vi "Step Association Retrieve Record.vi"(8 "error in (no error)":errorcluster, 11 "Statement Refnum":T1) -> (0 "error out":errorcluster, 2 "Association":T2, 3 "Statement Refnum":T1)   [LabVIEW 2011]
uses:
  Step Association Record.ctl
  SI.LIB/ODBC/SQL Controls/Statement Refnum.ctl
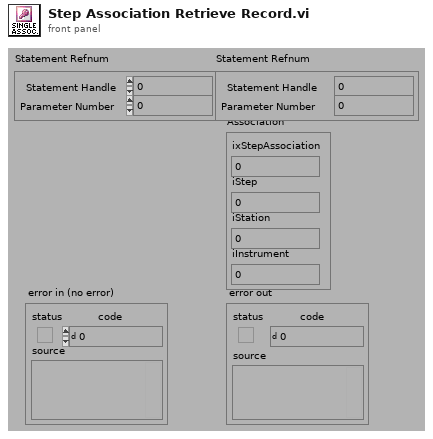
[diagram p1: front panel]
types:
  T1 = typedef "Statement Refnum.ctl" = cluster{"Statement Handle":i32, "Parameter Number":u16}
  T2 = typedef "Step Association Record.ctl" = cluster{"ixStepAssociation":i32, "iStep":i32, "iStation":i32, "iInstrument":i32}
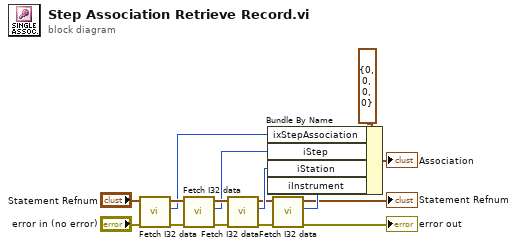
[diagram p0: block diagram]
diagram:
  n1 = call "Fetch I32 data.vi"("error in (no error)"="error in (no error)", "Statement Refnum"="Statement Refnum") -> ("error out"=w14:errorcluster, "Data"=w10:i32, "Statement Refnum"=w13:T1)  [unwired: 3 out]
  n2 = call "Fetch I32 data.vi"("error in (no error)"=w14, "Statement Refnum"=w13) -> ("error out"=w11:errorcluster, "Data"=w9:i32, "Statement Refnum"=w12:T1)  [unwired: 3 out]
  n3 = call "Fetch I32 data.vi"("error in (no error)"=w11, "Statement Refnum"=w12) -> ("error out"=w1:errorcluster, "Data"=w8:i32, "Statement Refnum"=w2:T1)  [unwired: 3 out]
  n4 = call "Fetch I32 data.vi"("error in (no error)"=w1, "Statement Refnum"=w2) -> ("error out"=→"error out":errorcluster, "Data"=w5:i32, "Statement Refnum"=→"Statement Refnum":T1)  [unwired: 3 out]
  n5 = Bundle By Name(cluster=T2 {"ixStepAssociation"=0, "iStep"=0, "iStation"=0, "iInstrument"=0} ("Step Association Record"), "ixStepAssociation"=w10, "iStep"=w9, "iStation"=w8, "iInstrument"=w5) -> (→"Association":T2)
